vi "DE_Map State into Bounds.vi"(6 "DE settings":T3={"population size"=10, "scale factor"=0.9, "crossover probability"=0.95, "bound mapping method"=1, "mutation method"=0, "crossover method"=0} {"crossover method" items=["Uniform", "Exponential"]; "mutation method" items=["Random", "Either Or", "Best", "Target to Best"]; "bound mapping method" items=["None", "Random between Bounds and Values", "Re-Initialize"]}, 7 "Bounds":cluster{"Min":dbl[], "Max":dbl[]}, 8 "error in (no error)":errorcluster, 9 "State In":T1, 10 "Base Indexes":i32[](array[numeric]), 11 "Candidate State In":T1) -> (0 "error out":errorcluster, 1 "State Out":T1, 3 "Candidate State Out":T1)   [LabVIEW 2017, in "NI_AAL_GlobalOptimization.lvlib"]
uses:
  <vilib>/gmath/NI_AAL_GlobalOptimization.lvlib
  <vilib>/gmath/GlobalOptimization.llb/DE_State.ctl
  <vilib>/gmath/GlobalOptimization.llb/DE_Population.ctl
  <vilib>/gmath/GlobalOptimization.llb/DE_Settings.ctl
  <vilib>/gmath/GlobalOptimization.llb/DE_Bound Mapping Method.ctl
  <vilib>/gmath/GlobalOptimization.llb/DE_Mutation Method.ctl
  <vilib>/gmath/GlobalOptimization.llb/DE_Crossover Method.ctl
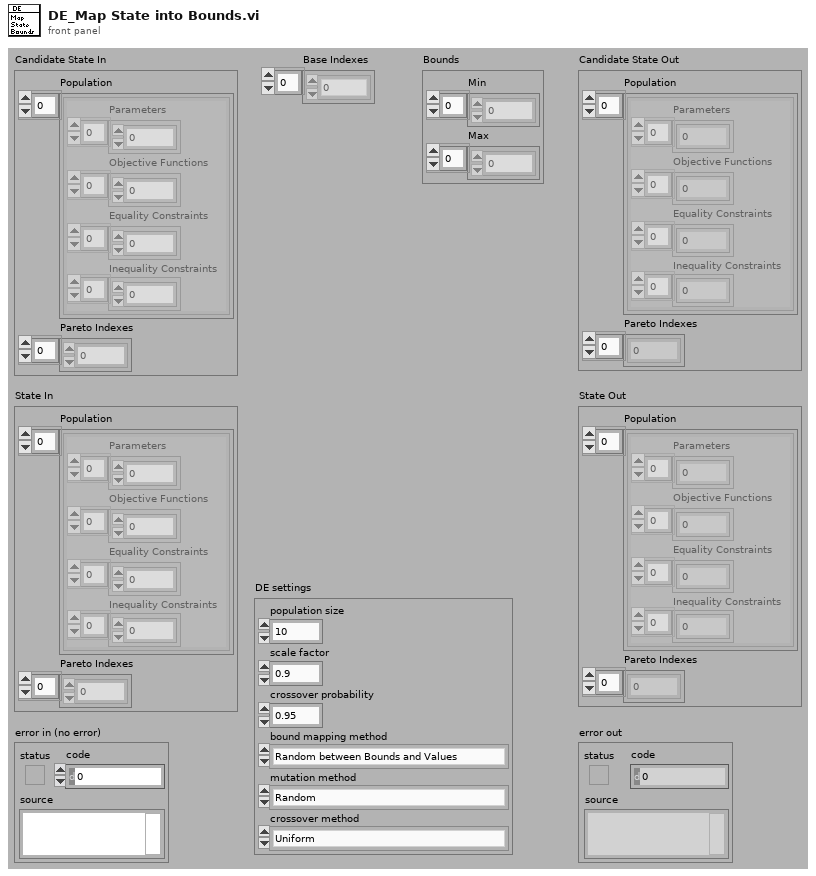
[diagram p1: front panel]
types:
  T1 = typedef "NI_AAL_GlobalOptimization.lvlib/DE_State.ctl" = cluster{"Population":T2[], "Pareto Indexes":i32[]}
  T2 = typedef "NI_AAL_GlobalOptimization.lvlib/DE_Population.ctl" = cluster{"Parameters":dbl[], "Objective Functions":dbl[], "Equality Constraints":dbl[], "Inequality Constraints":dbl[]}
  T3 = typedef "NI_AAL_GlobalOptimization.lvlib/DE_Settings.ctl" = cluster{"population size":i32, "scale factor":dbl, "crossover probability":dbl, "bound mapping method":T4, "mutation method":T5, "crossover method":T6}
  T4 = typedef "NI_AAL_GlobalOptimization.lvlib/DE_Bound Mapping Method.ctl" = u16
  T5 = typedef "NI_AAL_GlobalOptimization.lvlib/DE_Mutation Method.ctl" = u16
  T6 = typedef "NI_AAL_GlobalOptimization.lvlib/DE_Crossover Method.ctl" = u16
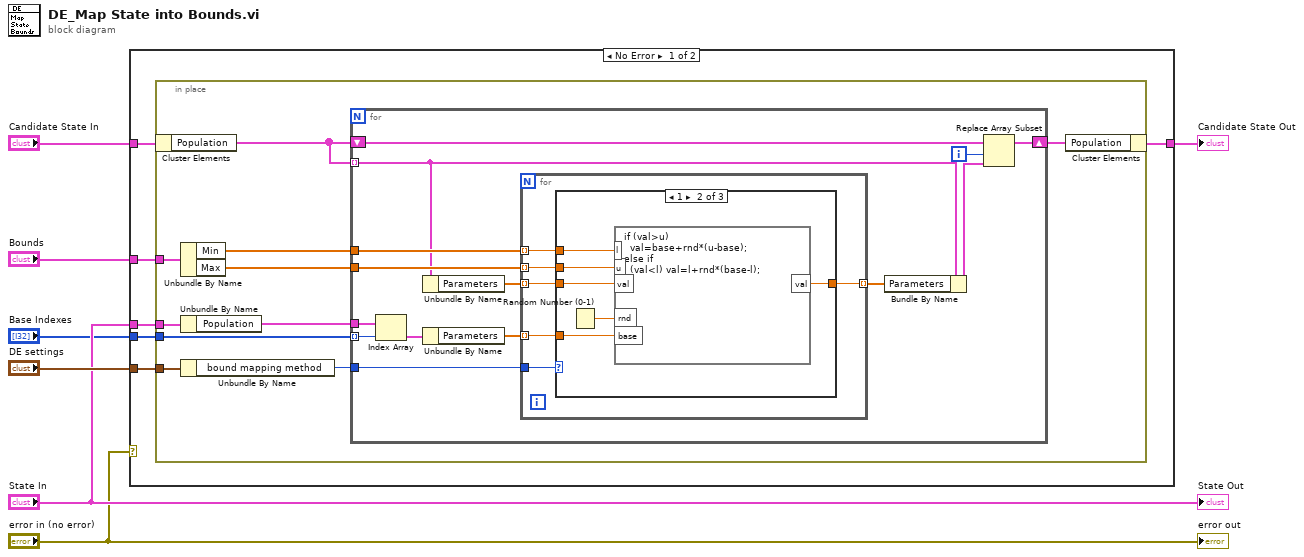
[diagram p0: block diagram]
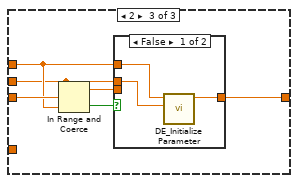
[diagram p3: hidden frame]
diagram:
  n1 = case shown="No Error" "error in (no error)" {
    tunnel: "DE settings" -> [w11 _]
    tunnel: "Bounds" -> [w12 _]
    tunnel: "Candidate State In" -> [w9 w61]
    tunnel: "State In" -> [w13 _]
    tunnel: [w8 w61] -> w4
    tunnel: "Base Indexes" -> [w10 _]
    frame No Error {
      n2 = in-place {
        in-place-border: w13 -> [w23]
        in-place-border: w12 -> [w20]
        in-place-border: w11 -> [w17]
        in-place-border: w10 -> [w16]
        n3 = in-place-cluster #1(w9) -> ("Population"=w15:T2[])
        n4 = Unbundle By Name(w20) -> ("Min"=w19:dbl[], "Max"=w18:dbl[])
        n5 = Unbundle By Name(w23) -> ("Population"=w22:T2[])
        n6 = Unbundle By Name(w17) -> ("bound mapping method"=w21:T4)
        n7 = for {
          tunnel: w15 -> [w25] mode=indexing
          tunnel: w22 -> [w37]
          tunnel: w21 -> [w33]
          shift-right: [w30] -> w14
          shift-left: w15 -> [w31]
          tunnel: w19 -> [w27]
          tunnel: w18 -> [w26]
          tunnel: w16 -> [w24] mode=indexing
          i -> [w28]
          n8 = Index Array(array=w37, index=w24) -> (element=w36:T2)
          n9 = Unbundle By Name(w25) -> ("Parameters"=w34:dbl[])
          n10 = Unbundle By Name(w36) -> ("Parameters"=w35:dbl[])
          n11 = for {
            tunnel: w35 -> [w38] mode=indexing
            tunnel: w34 -> [w42] mode=indexing
            tunnel: w33 -> [w43]
            tunnel: [w41] -> w32 mode=indexing
            tunnel: w27 -> [w40] mode=indexing
            tunnel: w26 -> [w39] mode=indexing
            n12 = case shown="1" w43 {
              tunnel: w42 -> [w44 w47 w53]
              tunnel: [w44 w46 w54] -> w41
              tunnel: w40 -> [_ w49 w52]
              tunnel: w39 -> [_ w48 w51]
              tunnel: w38 -> [_ w45 _]
              frame 0, Default {
              }
              frame 1 {
                n13 = Random Number (0-1)() -> (number: 0 to 1=w50:dbl)
                n14 = formula code="if (val>u)\n  val=base+rnd*(u-base);\nelse if\n  (val<l) val=l+rnd*(base-l);"("u"=w48, "l"=w49, "val"=w47, "rnd"=w50, "base"=w45) -> ("val"=w46:dbl)
              }
              frame 2 {
                n15 = In Range and Coerce(upper limit=w51, x=w53, lower limit=w52) -> (coerced(x)=w55:dbl, In Range?=w56:bool)
                n16 = case shown="False" w56 {
                  tunnel: [w59 w60] -> w54
                  tunnel: w55 -> [_ w60]
                  tunnel: w52 -> [w57 _]
                  tunnel: w51 -> [w58 _]
                  frame False {
                    n17 = call <vilib>:"DE_Initialize Parameter.vi"("max bound"=w58, "min bound"=w57) -> ("parameter"=w59:dbl)  [unwired: 9 in]
                  }
                  frame True {
                  }
                }
              }
            }
          }
          n18 = Bundle By Name(cluster=w25, "Parameters"=w32) -> (w29:T2)
          n19 = Replace Array Subset(array=w31, new element=w29, index=w28) -> (w30:T2[])
        }
        n20 = in-place-cluster #1("Population"=w14) -> (w8:T1)
      }
    }
    frame Error {
    }
  }
  "Candidate State Out" <- w4
  "State Out" <- "State In"
  "error out" <- "error in (no error)"
